vi "DAQ Control Functional Global.vi"(7 "State":T1, 8 "Error In":errorcluster, 10 "Processing Finished In":bool, 11 "DAQ Finished In":bool) -> (0 "Error Out":errorcluster, 1 "Reset?":bool, 2 "Processing Finished?":bool, 3 "DAQ Finished":bool)   [LabVIEW 2015]
uses:
  DAQ Control Functional Global States.ctl
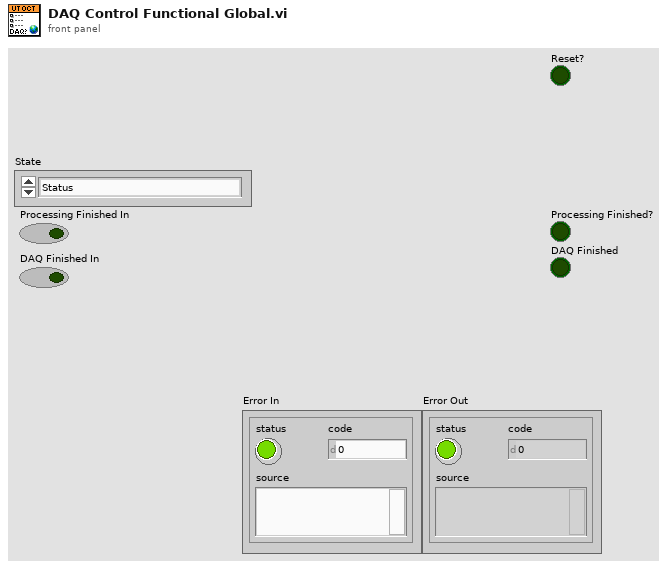
[diagram p1: front panel]
types:
  T1 = typedef "DAQ Control Functional Global States.ctl" = enum16{"Status", "Set Processing Finished", "Reset", "Clear", "Set DAQ Finished"}
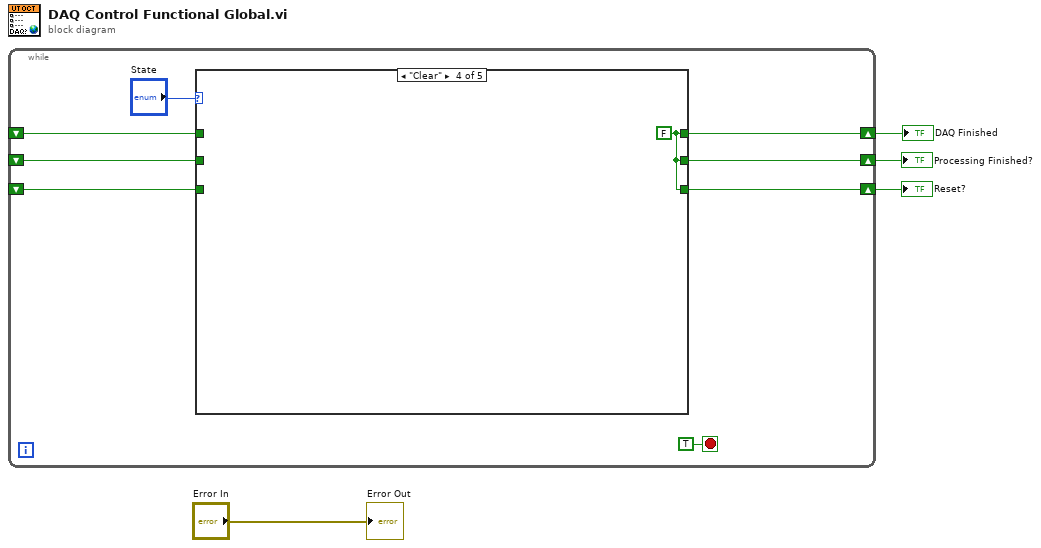
[diagram p0: block diagram]
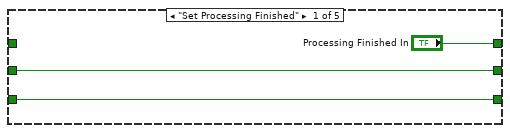
[diagram p2: hidden frame]
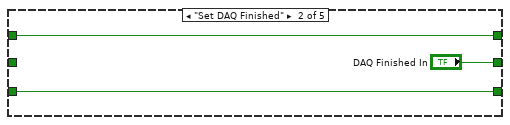
[diagram p3: hidden frame]
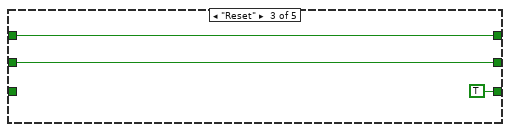
[diagram p4: hidden frame]
diagram:
  n1 = while {
    shift-right: [w9] -> w1
    shift-left: _ -> [w10]
    shift-right: [w7] -> w2
    shift-left: _ -> [w8]
    shift-right: [w5] -> w3
    shift-left: _ -> [w6]
    stop <- TRUE ("stop") stop-if-true
    n2 = case shown="\"Clear\"" "State" {
      tunnel: w10 -> [_ w18 w21 _ w25]
      tunnel: ["Processing Finished In" w18 w21 w22 w25] -> w9
      tunnel: w8 -> [w14 _ w20 _ w24]
      tunnel: [w14 "DAQ Finished In" w20 w22 w24] -> w7
      tunnel: w6 -> [w13 w16 _ _ w23]
      tunnel: [w13 w16 TRUE ("Processing Finished In") w22 w23] -> w5
      frame "Set Processing Finished" {
      }
      frame "Set DAQ Finished" {
      }
      frame "Reset" {
      }
      frame "Clear" {
        w22 = FALSE ("Processing Finished In")
      }
      frame "Status", Default {
      }
    }
  }
  "Processing Finished?" <- w2
  "DAQ Finished" <- w1
  "Reset?" <- w3
  "Error Out" <- "Error In"
